vi "editDialog.vi"(0 "reference in":refnum<class "DQMHModuleNode.lvclass">, 1 "insidePackageNode":bool, 5 "error in (no error)":errorcluster) -> (14 "reference out":refnum<class "DQMHModuleNode.lvclass">, 15 "changeConnection":T1, 16 "cancel":bool, 19 "error out":errorcluster)   [LabVIEW 2020, in "DQMHModuleNode.lvclass"]
doc: "Edit Dialog"
uses:
  <resource>/Framework/Providers/Open_GDS/UML/DQMHModuleNode_class/DQMHModuleNode.lvclass
  C:/Program Files (x86)/National Instruments/LabVIEW 2020/resource/Framework/Providers/Open_GDS/UML/AbstractNode_class/AbstractNode.lvclass
  <resource>/Framework/Providers/Open_GDS/UML/AbstractNode_class/private/NodeConnectionStatsType.ctl
  <resource>/Framework/Providers/Open_GDS/UML/UMLEditor/UMLEditor_StoredPathes.ctl
  <resource>/Framework/Providers/Open_GDS/UML/ContextHelp/ContextHelp_HelpTexts.ctl
  <vilib>/LabVIEW Icon API/lv_icon/Classes/Icon/Icon.lvclass
  <vilib>/LabVIEW Icon API/API_Text.ctl
  <vilib>/LabVIEW Icon API/API_Rectangle Colors.ctl
  <vilib>/LabVIEW Icon API/API_Rectangle Dimension.ctl
  <vilib>/LabVIEW Icon API/API_User Layer Data.ctl
  <vilib>/Utility/miscctls.llb/LVPoint32TypeDef.ctl
  <vilib>/picture/picture.llb/imagedata.ctl
  <vilib>/LabVIEW Icon API/API_Test Settings.ctl
  <vilib>/LabVIEW Icon API/lv_icon/Controls/Alignment.ctl
  <vilib>/LabVIEW Icon API/API_Text Colors.ctl
  <resource>/Framework/Providers/Open_GDS/UML/MultiLineString_class/MultiLineString.lvclass
  <resource>/Framework/Providers/Open_GDS/UML/AbstractNode_class/AbstractNode.lvclass
  <resource>/Framework/Providers/Open_GDS/UML/DQMH_API_class/DQMH_API.lvclass
  <vilib>/LabVIEW Icon API/LabVIEW Icon API.lvlib
panel:
  in  "ShowDescription":bool caption="Show Internal Data"
  out "ModuleIcon":picture caption="Library icon"
  in  "ModuleDescription":string caption="Module Description"
  in  "Template":u16(ring) items=["Singleton", "Cloneable"]
  out "RelText":string="Relative path used"
  in  "ShowInternalData":bool caption="Show Internal Data"
  in  "ShowEvents":bool caption="Show Events"
  in  "Help":bool
  in  "AddEvent":bool
  in  "AddInternalData":bool
  in  "Module Name":string
  in  "ModulePath":path caption="Library Path(Optional)"
  in  "InternalData":string caption="Internal Data"
  in  "Events":string
  in  "connection":bool caption="Disconnect from Package"
  in  "Cancel Button":bool
  in  "OK Button":bool
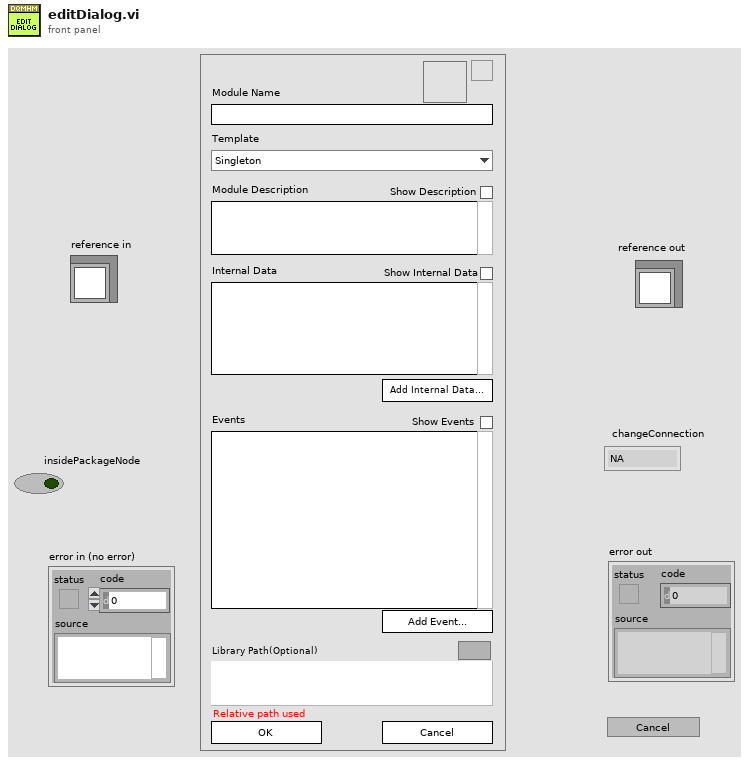
[diagram p1: front panel]
types:
  T1 = typedef "AbstractNode.lvclass/NodeConnectionStatsType.ctl" = enum16{"NA", "Connect", "DisConnect"}
  T2 = cluster{"Cancelled":bool, "Event":refnum<event-registration>, "changeConnection":T1, "Icon":u8[][], "NameModifed":bool}
  T3 = typedef "UMLEditor_StoredPathes.ctl" = enum16{"LastSearchPath", "QueuedArrayStateVI", "ClassBasePath", "ViTemplatePath", "ApplicationTemplatePath", "IniFilePath", "WizDir", "RevPlugInPath"}
  T4 = cluster{"left":i16, "top":i16, "right":i16, "bottom":i16}
  T5 = cluster{"Selection Start":u32, "Selection End":u32}
  T6 = cluster{"LibraryIcon":string, "HeaderRows(1)":u8}
  T7 = typedef "ContextHelp_HelpTexts.ctl" = enum16{"None(Hide)", "Default", "Help", "Welcome", "GettingStarted", "ClassDiagram_Help", "SequenceDiagram_Help", "UseCaseDiagram_Help", "BSelect", "BClass", "BInterface", "BPackage", "BNote", "BDependency", "BInheritance", "BInterfaceImplementation", "BAssociation", "BAggregation", "BCompAggregation", "BNoteConnector", "BObject", "BActionBar", "BCall", "BSystem", "BActor", "BUseCase", "BGeneralization", "BIncludes", "BExtends", "BUseCaseDiagramAssociation", "ClassRelationshipEdge editDialog_Bent Style", "ClassRelationshipEdge editDialog_RelationType", "ClassRelationshipEdge editDialog_Reverse association", "ClassRelationshipEdge editDialog_Start label", "ClassRelationshipEdge editDialog_Middle label", "ClassRelationshipEdge editDialog_End label", "UMLEditor reversedEngineering_Pathes", "ReversedEngineering StateReverseDialog_Help", "ReversedEngineering StateQueuedSettings_Help", "UMLEditor reversedEngineering_AddTopVIs", "UMLEditor reversedEngineering_AddClasses", "UMLEditor reversedEngineering_AddDirs", "UMLEditor reversedEngineering_Recursively", "UMLEditor reversedEngineering_Remove", "UMLEditor reversedEngineering_ClearList", "UMLEditor reversedEngineering_HideSubAss", "UMLEditor reversedEngineering_CreateTypes", "UMLEditor reversedEngineering_OnlyInheritance", "UMLEditor reversedEngineering_CreateApplication", "UMLEditor reversedEngineering_OK", "UMLEditor reversedEngineering_Cancel", "UMLEditor reversedEngineering_Help", "UMLEditor createWizardScriptFile_ScriptfilePath", "UMLEditor createWizardScriptFile_ClassPath", "UMLEditor createWizardScriptFile_Use", "UMLEditor createWizardScriptFile_PrivateDirName", "UMLEditor createWizardScriptFile_DirAppend", "UMLEditor createWizardScriptFile_Separator Character", "UMLEditor createWizardScriptFile_OK", "UMLEditor createWizardScriptFile_Cancel", "UMLEditor createWizardScriptFile_Help", "ClassNode editDialog_Class Name", "InterfaceNode editDialog_Class Name", "ClassNode editDialog_Attribute", "ClassNode editDialog_Methods", "InterfaceNode editDialog_Methods", "ClassNode editDialog_connection", "InterfaceNode editDialog_connection", "ClassNode editDialog_StereoType", "ClassNode editDialog_ShowAttrib", "ClassNode editDialog_ShowMethods", "ClassNode editDialog_ClassPath", "ClassNode editDialog_AddAttribute", "ClassNode editDialog_AddMethod", "InterfaceNode editDialog_AddMethod", "ClassNode AttributeGuide_AttributeName", "ClassNode AttributeGuide_Array?", "ClassNode AttributeGuide_Data Type", "ClassNode AttributeGuide_RefName", "ClassNode AttributeGuide_Preview", "ClassNode AttributeGuide_OK", "ClassNode AttributeGuide_Cancel", "ClassNode MethodGuide_Visibility", "ClassNode MethodGuide_Method Name", "ClassNode MethodGuide_Preview", "ClassNode MethodGuide_OK", "ClassNode MethodGuide_Cancel", "CallNode EditCallProperties_AllButtons", "ObjectNode EditObjectlProperties_AllButtons", "ActorNode EditActorProperties_AllButtons", "UseCaseRelationshipNode EditUseCaselProperties_AllButtons", "UseCaseNode EditUseCaselProperties_AllButtons", "SystemNode EditSystemProperties_AllButtons", "ReversedEngineering UpdateAttributes_AllButtons", "StateNode editDialog_AllButtons", "StateTransition editDialog_AllButtons", "ArrangeNodes Main_Picture", "ArrangeNodes Main_Zoom", "ArrangeNodes Main_Auto Zoom", "ArrangeNodes Main_shorten", "ArrangeNodes Main_Min Length", "ArrangeNodes Main_Max Length", "ArrangeNodes Main_increase", "ArrangeNodes Main_decrease", "ArrangeNodes Main_Shake", "ArrangeNodes Main", "BState", "BInitialState", "BFinalState", "BStateTransition", "StateDiagram_Help", "StateDiagram_PropertiesAllButtons", "ReversedEngineering StateReverseDialog_ClearStates", "ReversedEngineering StateReverseDialog_UseQueuedStateMachines", "ReversedEngineering StateReverseDialog_QueuedSettings", "ReversedEngineering StateReverseDialog_SearchForVIs", "ReversedEngineering StateReverseDialog_SearchCriteria", "OptionsDialog_ClassBasePath", "OptionsDialog_VIPath", "OptionsDialog_ApplicationPath", "OptionsDialog_WizDir", "OptionsDialog_IniFilePath", "OptionsDialog_DefineColors", "OptionsDialog_Help", "OptionsDialog_CreateTypes", "ClassRelationshipEdge editDialog_SplitWire"}
  T8 = typedef "LabVIEW Icon API.lvlib/API_Test Settings.ctl" = cluster{"Font":string, "Alignment":T9, "Size":u8, "Center text":bool, "Capitalize text":bool, "Text color":T10}
  T9 = typedef "Alignment.ctl" = u16
  T10 = typedef "LabVIEW Icon API.lvlib/API_Text Colors.ctl" = cluster{"Line 1 color":u32, "Line 2 color":u32, "Line 3 color":u32, "Line 4 color":u32}
  T11 = typedef "LabVIEW Icon API.lvlib/API_User Layer Data.ctl" = cluster{"Layer name":string, "Origin":T12, "Icon image data":T13}
  T12 = typedef "LVPoint32TypeDef.ctl" = cluster{"Horizontal":i32, "Vertical":i32}
  T13 = typedef "imagedata.ctl" = cluster{"image type":i32, "image depth":i32, "image":u8[], "mask":u8[], "colors":u32[], "Rectangle":cluster{"left":i16, "top":i16, "right":i16, "bottom":i16}}
  T14 = typedef "LabVIEW Icon API.lvlib/API_Rectangle Dimension.ctl" = cluster{"Width":i16, "Height":i16}
  T15 = typedef "LabVIEW Icon API.lvlib/API_Rectangle Colors.ctl" = cluster{"Border":u32, "Background":u32}
  T16 = typedef "LabVIEW Icon API.lvlib/API_Text.ctl" = cluster{"Line 1 text":string, "Line 2 text":string, "Line 3 text":string, "Line 4 text":string}
  T17 = typedef "DQMHModuleNode.lvclass/ObjectAttributes.ctl" = cluster{"DescriptionHeight":dbl, "InternalDataHeight":dbl, "EventsHeight":dbl, "Name":refnum<class "MultiLineString.lvclass">, "Description":refnum<class "MultiLineString.lvclass">, "InternalData":refnum<class "MultiLineString.lvclass">, "Events":refnum<class "MultiLineString.lvclass">, "showDescription":bool, "showInternalData":bool, "showEvents":bool, "DEFAULT_ROUNDING":i32, "DEFAULT_WIDTH":i32, "DEFAULT_HEIGHT":i32, "ClassPath":path, "Template":string, "Icon":u8[][]}
  T18 = typedef "AbstractNode.lvclass/ObjectAttributes.ctl" = cluster{"parent":refnum<class "AbstractNode.lvclass">, "children":refnum<class "AbstractNode.lvclass">[], "Hidden":bool}
  T19 = typedef "ContextHelp_ShowType.ctl" = cluster{"Header":string, "Picture":picture, "Text":string}
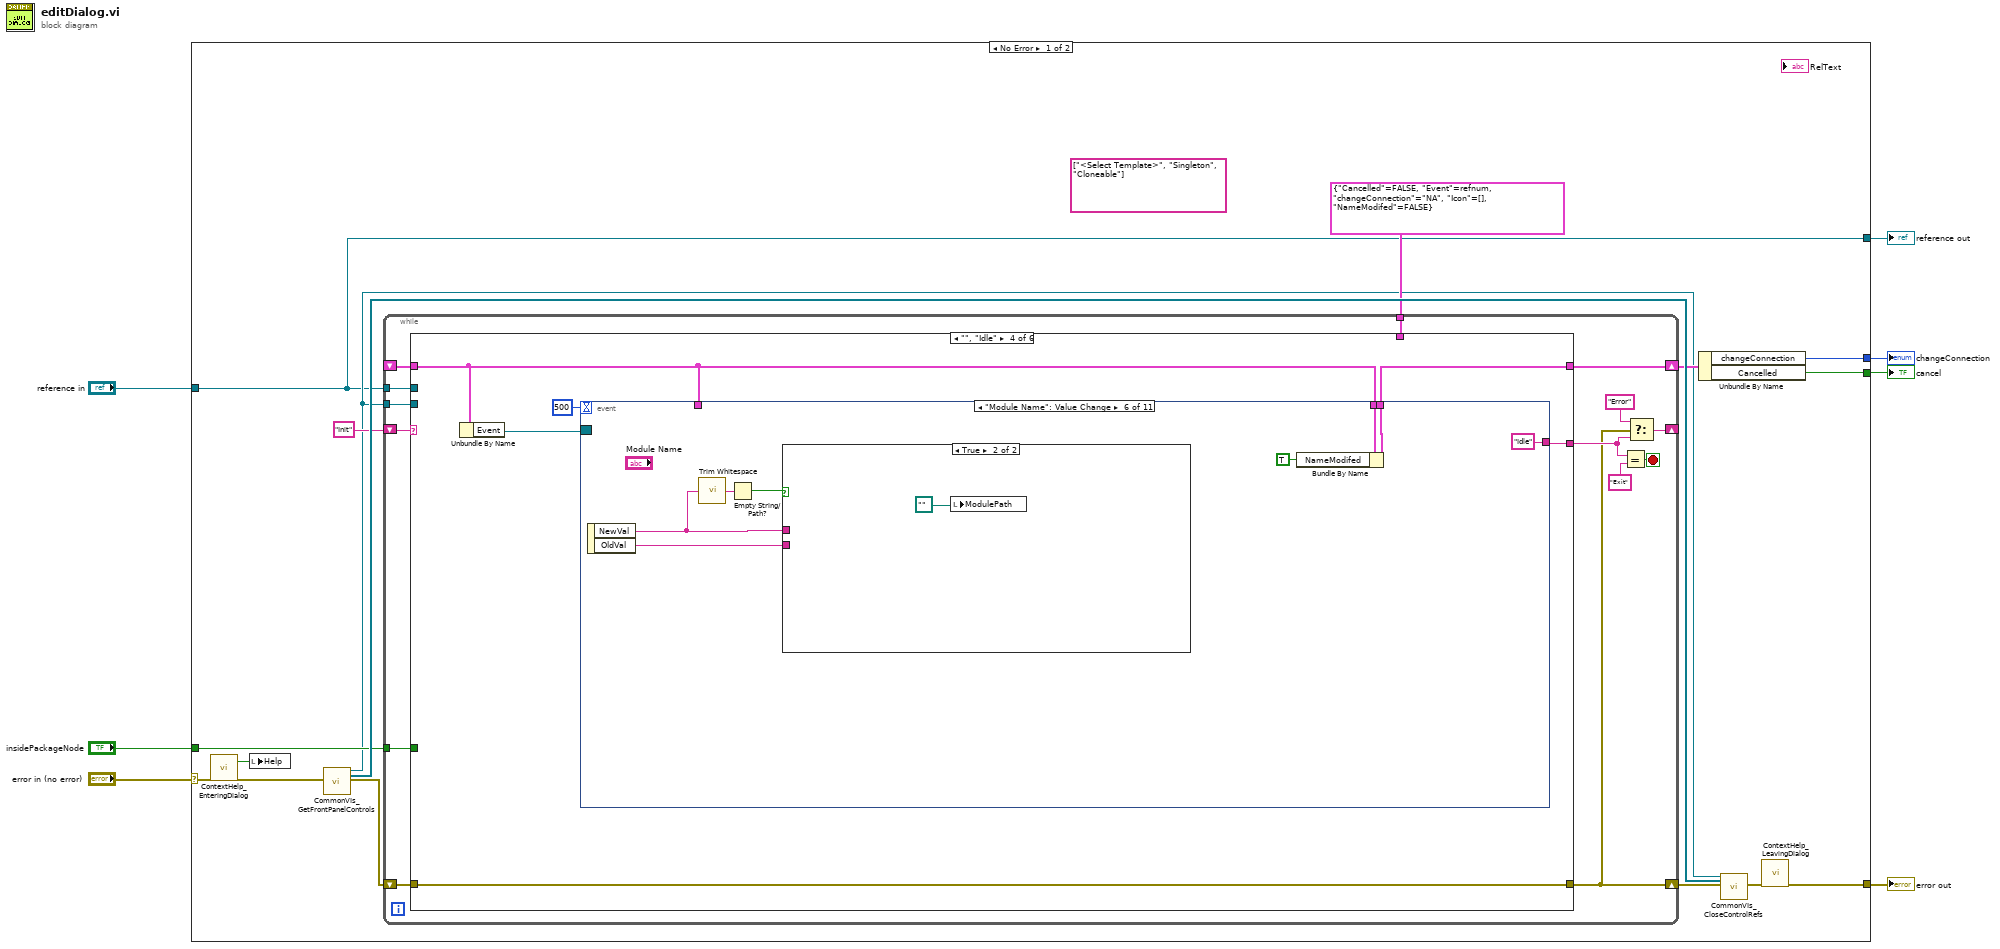
[diagram p0: block diagram]
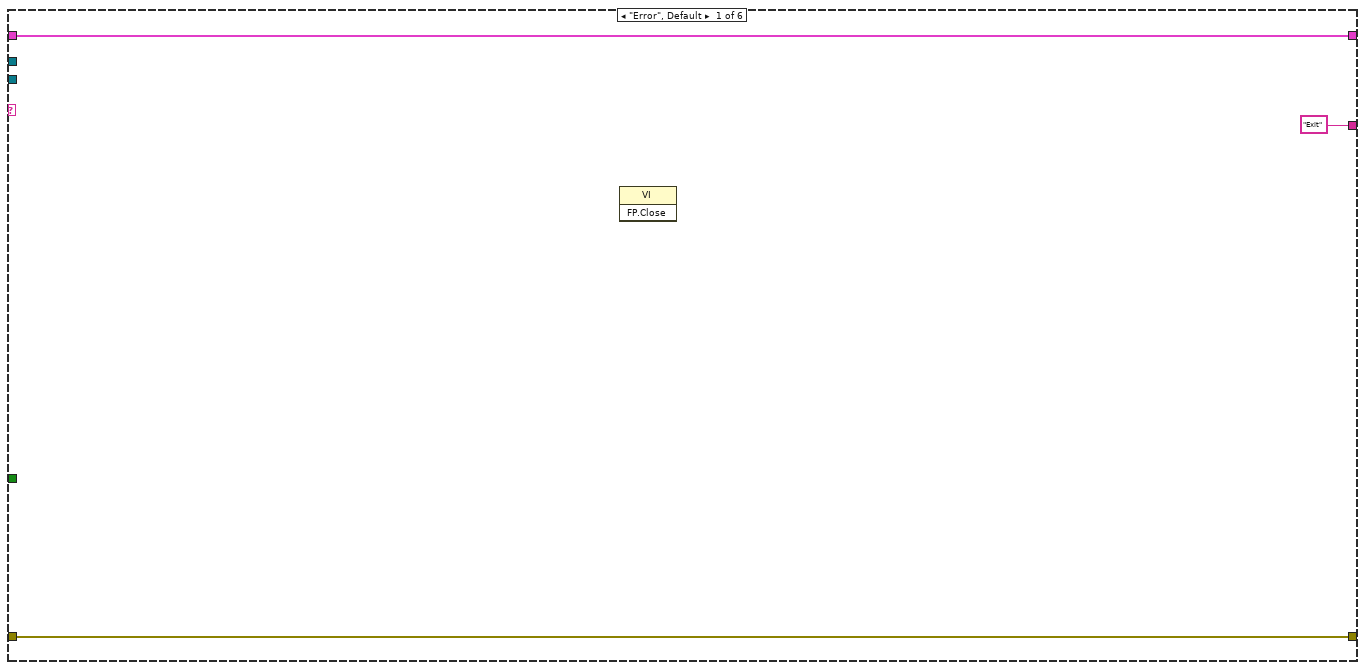
[diagram p2: hidden frame]
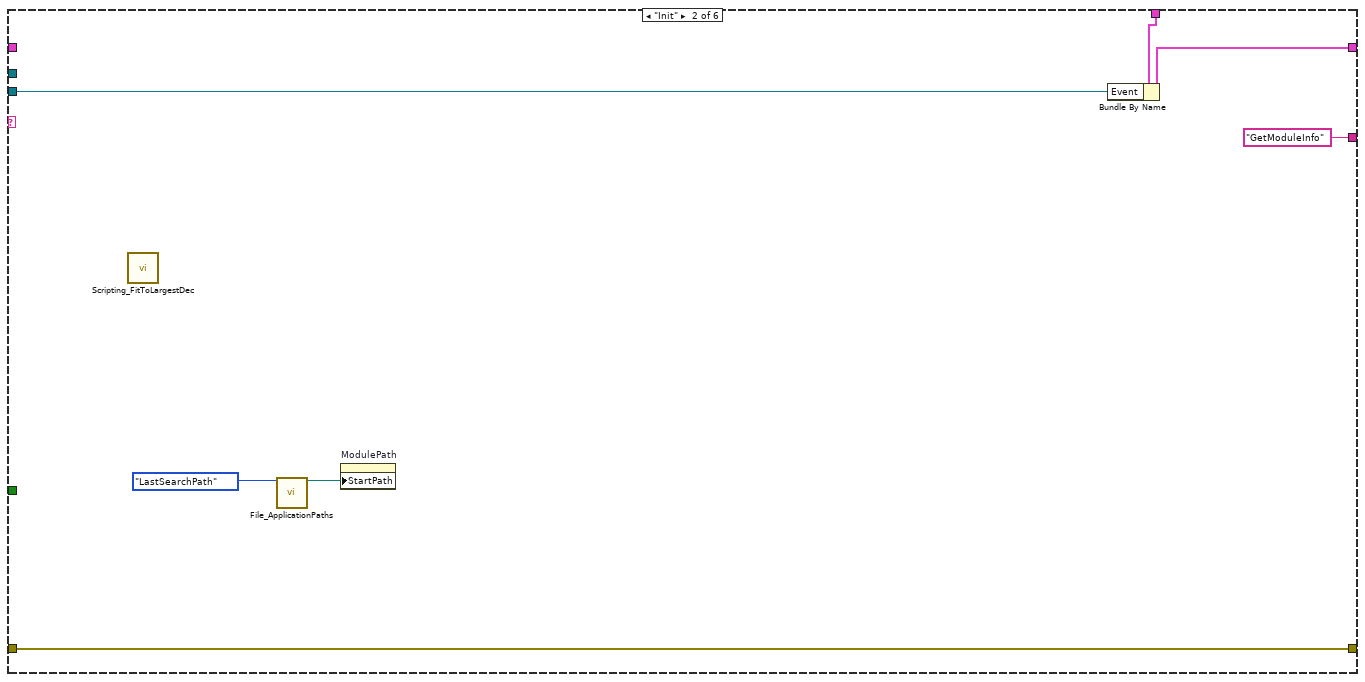
[diagram p3: hidden frame]
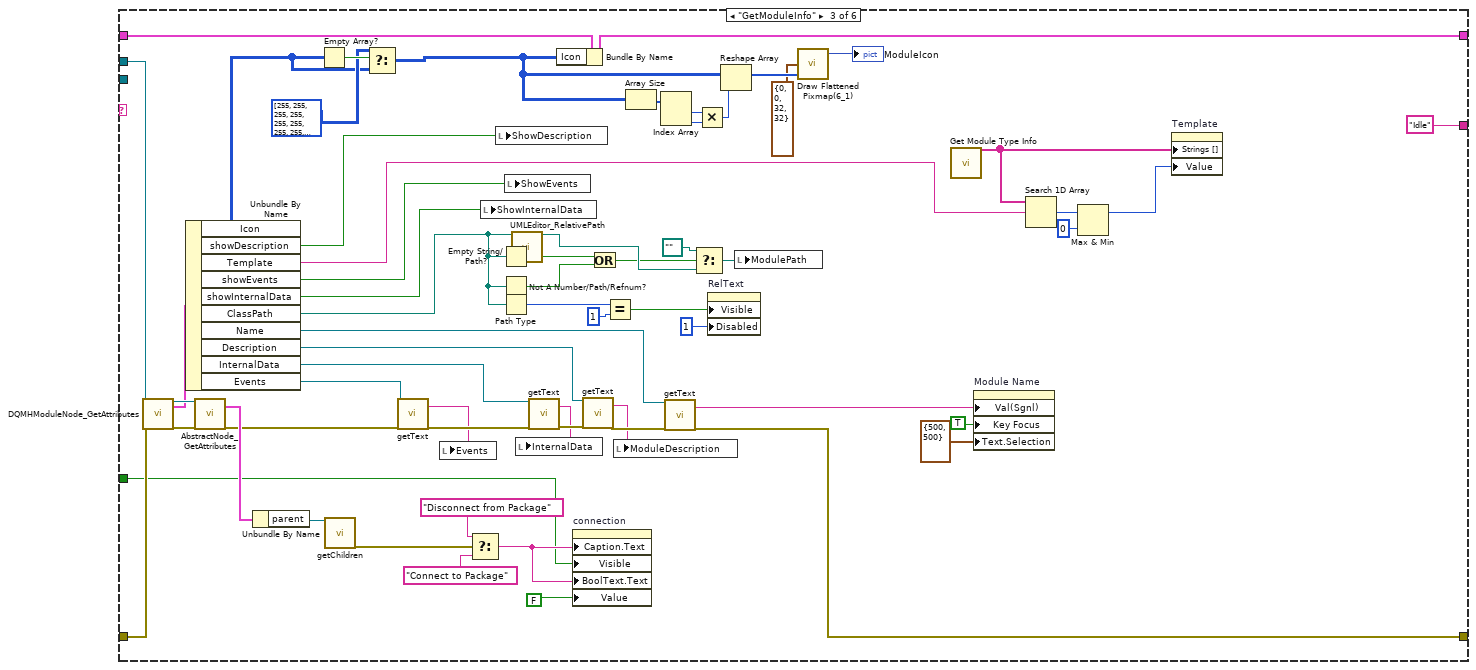
[diagram p4: hidden frame]
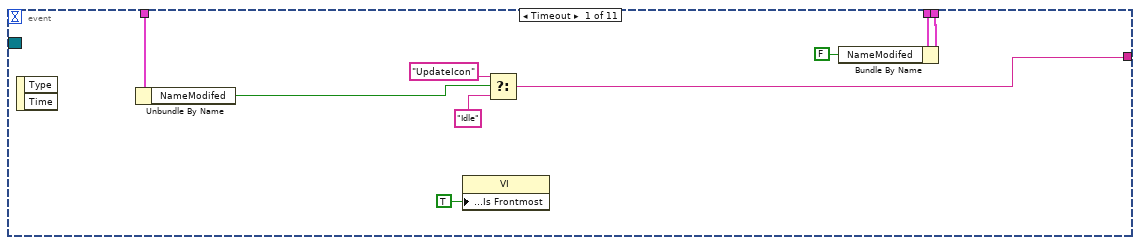
[diagram p5: hidden frame]
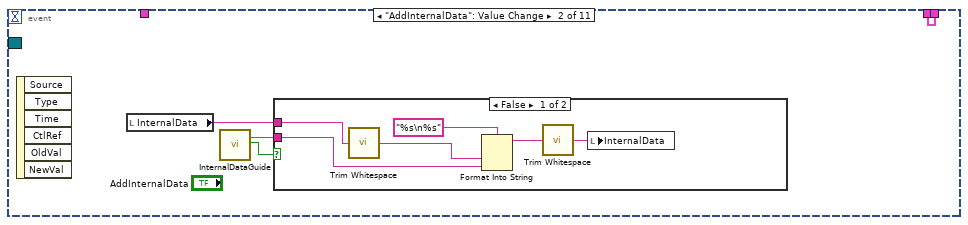
[diagram p6: hidden frame]
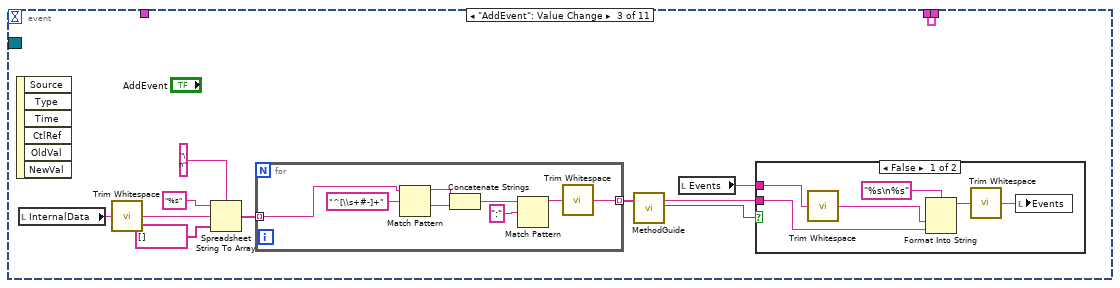
[diagram p8: hidden frame]
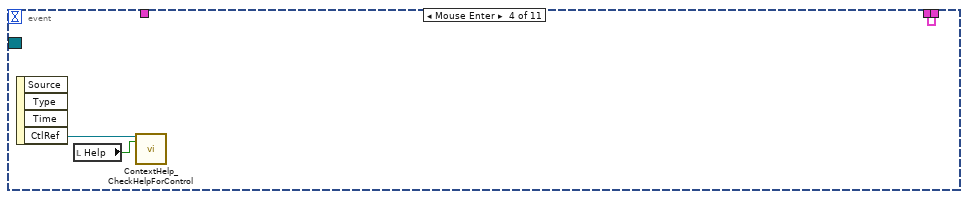
[diagram p10: hidden frame]
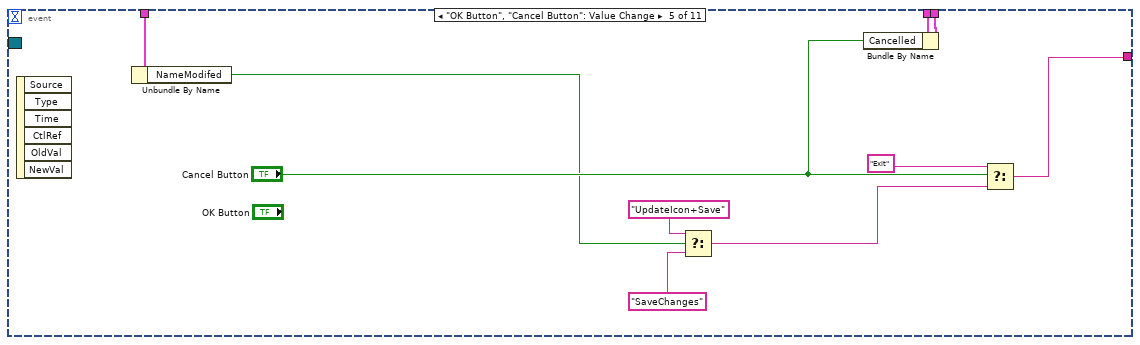
[diagram p11: hidden frame]
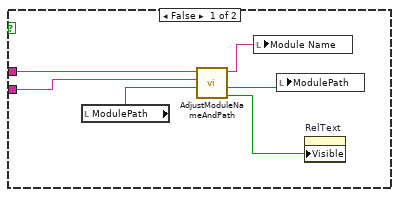
[diagram p12: hidden frame]
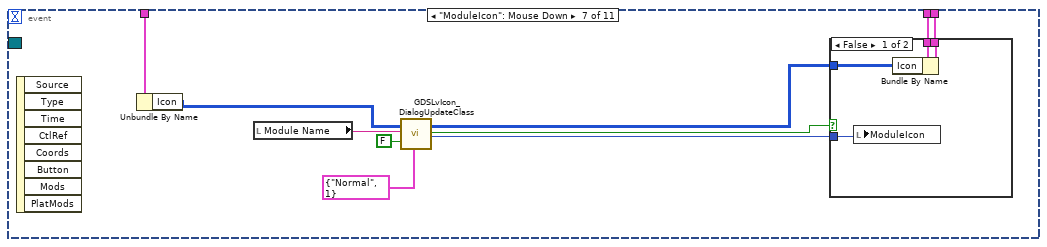
[diagram p13: hidden frame]
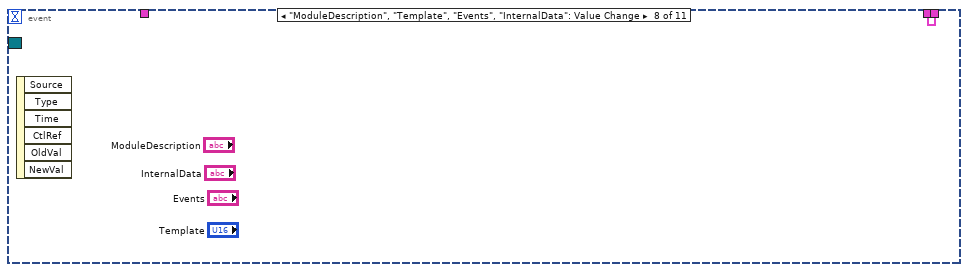
[diagram p15: hidden frame]
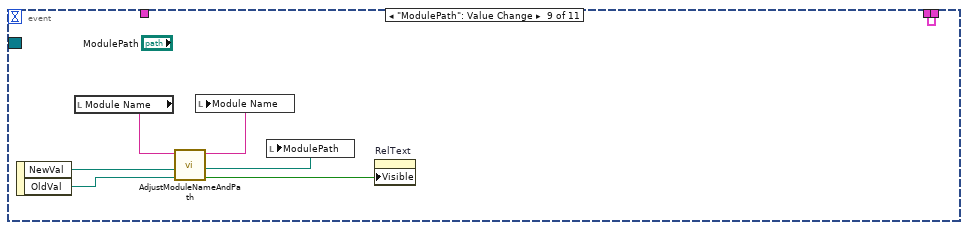
[diagram p16: hidden frame]
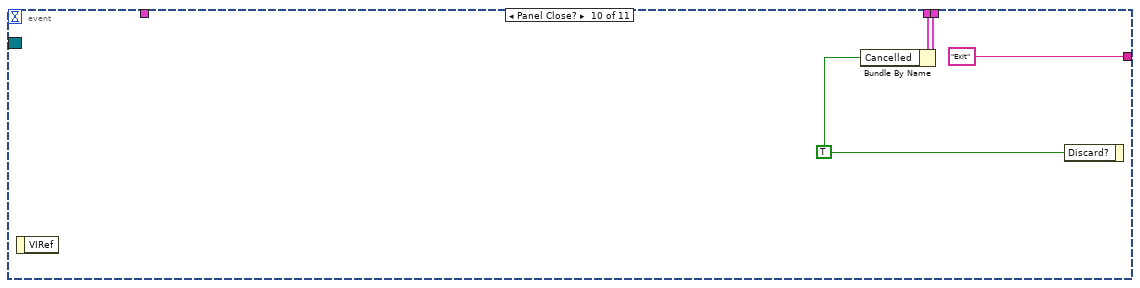
[diagram p17: hidden frame]
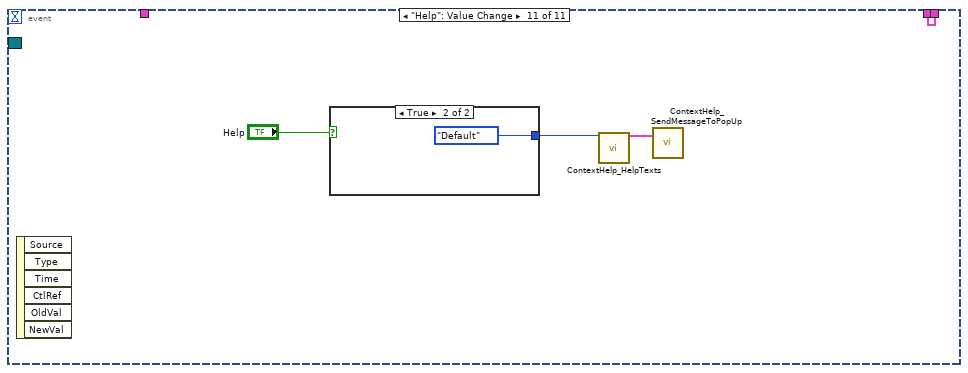
[diagram p18: hidden frame]
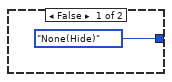
[diagram p19: hidden frame]
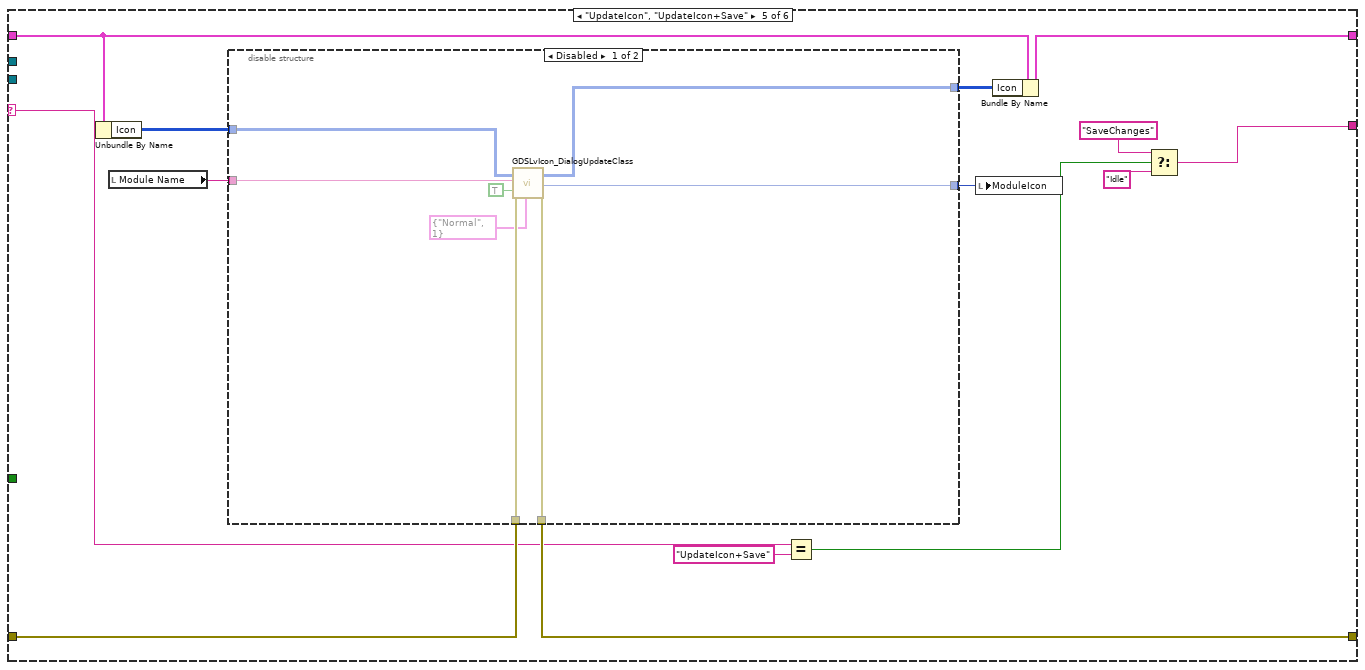
[diagram p20: hidden frame]
diagram:
  n1 = case shown="No Error" "error in (no error)" {
    selector: "error in (no error)" -> [w16 w312]
    tunnel: "reference in" -> [w8 w313]
    tunnel: [w13 w312] -> w5
    tunnel: [w8 w313] -> w4
    tunnel: "insidePackageNode" -> [w17 _]
    tunnel: [w10 _] -> w2
    tunnel: [w9 TRUE ("Key Focus")] -> w1
    frame No Error {
      (unwired) string[] ["<Select Template>", "Singleton", "Cloneable"] ("Strings []")
      n2 = call <resource>:"ContextHelp_EnteringDialog.vi"("error in (no error)"=w16) -> ("HelpStatus"=w23:bool, "error out"=w20:errorcluster)  [unwired: 2 in, 15 out]
      n3 = local write "Help"(w23) -> ()
      n4 = call <resource>:"CommonVIs_GetFrontPanelControls.vi"("error in (no error)"=w20) -> ("Event Registration Refnum"=w11:refnum<event-registration>, "ControlRefs"=w22:refnum<vi>[], "error out"=w15:errorcluster)  [unwired: 1 in, 15 out]
      n5 = while {
        shift-right: [w30] -> w14
        shift-left: w15 -> [w37]
        shift-right: [w35] -> _
        shift-left: "Init" -> [w36]
        shift-right: [w29] -> w12
        shift-left: _ -> [w28]
        tunnel: T2 {"Cancelled"=FALSE, "Event"=refnum, "changeConnection"=enum."NA", "Icon"=[], "NameModifed"=FALSE} -> [w27]
        tunnel: w17 -> [w26]
        tunnel: w11 -> [w25]
        tunnel: w8 -> [w24]
        stop <- w34 stop-if-true
        n6 = case shown="\"\", \"Idle\"" w36 {
          selector: w36 -> [_ _ _ _ w225 _]
          tunnel: w37 -> [w40 w46 w102 w112 w231 w276]
          tunnel: [w40 w46 w69 w112 w232 w266] -> w30
          tunnel: ["Exit" "GetModuleInfo" "Idle" w113 w221 "Exit"] -> w31
          tunnel: [w38 w45 w61 w114 w227 w280] -> w29
          tunnel: w28 -> [w38 _ w108 w109 w230 w261]
          tunnel: w27 -> [_ w44 _ _ _ _]
          tunnel: w26 -> [_ _ w95 _ _ w278]
          tunnel: w25 -> [_ w42 _ _ _ _]
          tunnel: w24 -> [_ _ w81 _ _ w281]
          frame "Error", Default {
            n7 = invoke class="VI" method="FP.Close"() -> ()  [unwired: 3 in, 3 out]
          }
          frame "Init" {
            n8 = call <resource>:"Scripting_FitToLargestDec.vi"() -> ()  [unwired: 6 in, 2 out]
            n9 = call <resource>:"File_ApplicationPaths.vi"("PathName"=UMLEditor_StoredPathes."LastSearchPath" ("UMLPathes")) -> ("Path Out"=w43:path)  [unwired: 3 in, 15 out]
            n10 = property on="ModulePath" class="Path"("StartPath"=w43) -> ()  [unwired: 2 in, 2 out]
            n11 = Bundle By Name(cluster=w44, "Event"=w42) -> (w45:T2)
          }
          frame "GetModuleInfo" {
            n12 = call <resource>:"DQMHModuleNode_GetAttributes.vi"("reference in"=w81, "error in (no error)"=w102) -> ("reference out"=w104:refnum<class "DQMHModuleNode.lvclass">, "Data"=w100:T17, "error out"=w103:errorcluster)  [unwired: 1 in, 14 out]
            n13 = Unbundle By Name(w100) -> ("Icon"=w58:u8[][], "showDescription"=w49:bool, "Template"=w66:string, "showEvents"=w84:bool, "showInternalData"=w83:bool, "ClassPath"=w82:path, "Name"=w99:refnum<class "MultiLineString.lvclass">, "Description"=w98:refnum<class "MultiLineString.lvclass">, "InternalData"=w97:refnum<class "MultiLineString.lvclass">, "Events"=w74:refnum<class "MultiLineString.lvclass">)
            n14 = call <resource>:"AbstractNode_GetAttributes.vi"("reference in"=w104, "error in (no error)"=w103) -> ("Data"=w101:T18, "error out"=w70:errorcluster)  [unwired: 14 in, 2 out]
            n15 = Unbundle By Name(w101) -> ("parent"=w68:refnum<class "AbstractNode.lvclass">)
            n16 = Empty Array?(array=w58) -> (empty?=w60:bool)
            n17 = call-dynamic "getChildren.vi"("reference"=w68) -> ("error out"=w67:errorcluster)  [unwired: 15 in, 3 out]
            n18 = Select(t=u8[][] [[255, 255, 255, 255, 255, 255, 255, 255, 255, 255, 255, 255, 255, 255, 255, 255, 255, 255, 255, 255, 255, 255, 255, 255, 255, 255, 255, 255, 255, 255, 255, 255], [255, 5, 5, 5, 5, 5, 5, 5, 5, 5, 5, 5, 5, 5, 5, 5, 5, 5, 5, 5, 5, 5, 5, 5, 5, 5, 5, 5, 5, 5, 5, 255], [255, 5, 5, 5, 5, 5, 255, 255, 255, 5, 5, 5, 255, 255, 5, 5, 255, 5, 5, 5, 255, 5, 255, 5, 5, 255, 5, 5, 5, 5, 5, 255], [255, 5, 5, 5, 5, 5, 255, 5, 5, 255, 5, 255, 5, 5, 255, 5, 255, 255, 5, 255, 255, 5, 255, 5, 5, 255, 5, 5, 5, 5, 5, 255], [255, 5, 5, 5, 5, 5, 255, 5, 5, 255, 5, 255, 5, 5, 255, 5, 255, 5, 255, 5, 255, 5, 255, 255, 255, 255, 5, 5, 5, 5, 5, 255], [255, 5, 5, 5, 5, 5, 255, 5, 5, 255, 5, 255, 5, 255, 5, 5, 255, 5, 5, 5, 255, 5, 255, 5, 5, 255, 5, 5, 5, 5, 5, 255], [255, 5, 5, 5, 5, 5, 255, 255, 255, 5, 5, 5, 255, 5, 255, 5, 255, 5, 5, 5, 255, 5, 255, 5, 5, 255, 5, 5, 5, 5, 5, 255], [255, 5, 5, 5, 5, 5, 5, 5, 5, 5, 5, 5, 5, 5, 5, 5, 5, 5, 5, 5, 5, 5, 5, 5, 5, 5, 5, 5, 5, 5, 5, 255], [255, 255, 255, 255, 255, 255, 255, 255, 255, 255, 255, 255, 255, 255, 255, 255, 255, 255, 255, 255, 255, 255, 255, 255, 255, 255, 255, 255, 255, 255, 255, 255], [255, 156, 156, 156, 156, 156, 156, 156, 156, 156, 156, 156, 156, 156, 156, 156, 156, 156, 156, 156, 156, 156, 156, 156, 156, 156, 156, 156, 156, 156, 156, 255], [255, 156, 156, 156, 156, 156, 156, 156, 156, 156, 156, 156, 156, 156, 156, 5, 5, 156, 156, 156, 156, 156, 156, 156, 156, 156, 156, 156, 156, 156, 156, 255], [255, 156, 156, 156, 156, 156, 156, 156, 156, 156, 156, 156, 156, 5, 89, 47, 89, 89, 5, 156, 156, 156, 156, 156, 156, 156, 156, 156, 156, 156, 156, 255], [255, 156, 156, 156, 156, 156, 156, 156, 156, 156, 156, 5, 89, 47, 5, 5, 5, 5, 89, 89, 5, 156, 156, 156, 156, 156, 156, 156, 156, 156, 156, 255], [255, 156, 156, 156, 156, 156, 156, 156, 156, 5, 89, 47, 5, 5, 5, 5, 5, 5, 5, 5, 89, 89, 5, 156, 156, 156, 156, 156, 156, 156, 156, 255], [255, 156, 156, 156, 156, 156, 156, 156, 89, 47, 5, 5, 5, 5, 5, 5, 5, 5, 5, 5, 5, 5, 89, 89, 156, 156, 156, 156, 156, 156, 156, 255], [255, 156, 156, 156, 156, 156, 156, 156, 47, 47, 5, 5, 5, 5, 5, 5, 5, 5, 5, 5, 5, 5, 173, 89, 156, 156, 156, 156, 156, 156, 156, 255], [255, 156, 156, 156, 156, 156, 156, 156, 47, 89, 89, 47, 5, 5, 5, 5, 5, 5, 5, 5, 173, 173, 173, 47, 156, 156, 156, 156, 156, 156, 156, 255], [255, 156, 156, 156, 156, 156, 156, 156, 47, 89, 89, 89, 89, 47, 5, 5, 5, 5, 173, 173, 173, 173, 173, 47, 156, 156, 156, 156, 156, 156, 156, 255], [255, 156, 156, 156, 156, 156, 156, 156, 47, 89, 89, 89, 89, 89, 89, 47, 89, 173, 173, 173, 173, 173, 173, 47, 156, 156, 156, 156, 156, 156, 156, 255], [255, 156, 156, 156, 156, 156, 156, 156, 47, 89, 89, 89, 89, 89, 89, 89, 173, 173, 173, 173, 173, 173, 173, 47, 156, 156, 156, 156, 156, 156, 156, 255], [255, 156, 156, 156, 156, 156, 156, 156, 47, 89, 89, 89, 89, 89, 89, 89, 173, 173, 173, 173, 173, 173, 173, 47, 156, 156, 156, 156, 156, 156, 156, 255], [255, 156, 156, 156, 156, 156, 156, 156, 47, 89, 89, 89, 89, 89, 89, 89, 173, 173, 173, 173, 173, 173, 173, 47, 156, 156, 156, 156, 156, 156, 156, 255], [255, 156, 156, 156, 156, 156, 156, 156, 47, 89, 89, 89, 89, 89, 89, 89, 173, 173, 173, 173, 173, 173, 173, 47, 156, 156, 156, 156, 156, 156, 156, 255], [255, 156, 156, 156, 156, 156, 156, 156, 47, 89, 89, 89, 89, 89, 89, 89, 173, 173, 173, 173, 173, 173, 173, 47, 156, 156, 156, 156, 156, 156, 156, 255], [255, 156, 156, 156, 156, 156, 156, 156, 89, 89, 89, 89, 89, 89, 89, 89, 173, 173, 173, 173, 173, 173, 89, 89, 172, 172, 172, 156, 156, 156, 156, 255], [255, 156, 156, 156, 156, 156, 156, 156, 156, 47, 47, 89, 89, 89, 89, 89, 173, 173, 173, 173, 89, 89, 47, 172, 172, 172, 172, 172, 172, 156, 156, 255], [255, 156, 156, 156, 156, 156, 156, 156, 156, 156, 156, 47, 89, 89, 89, 89, 173, 173, 89, 89, 47, 172, 172, 172, 172, 172, 172, 156, 156, 156, 156, 255], [255, 156, 156, 156, 156, 156, 156, 156, 156, 156, 156, 156, 156, 47, 89, 89, 89, 89, 5, 172, 172, 172, 172, 172, 172, 172, 156, 156, 156, 156, 156, 255], [255, 156, 156, 156, 156, 156, 156, 156, 156, 156, 156, 156, 156, 156, 156, 47, 5, 172, 172, 172, 172, 172, 172, 172, 156, 156, 156, 156, 156, 156, 156, 255], [255, 156, 156, 156, 156, 156, 156, 156, 156, 156, 156, 156, 156, 156, 156, 156, 156, 156, 172, 172, 172, 172, 156, 156, 156, 156, 156, 156, 156, 156, 156, 255], [255, 156, 156, 156, 156, 156, 156, 156, 156, 156, 156, 156, 156, 156, 156, 156, 156, 156, 156, 156, 156, 156, 156, 156, 156, 156, 156, 156, 156, 156, 156, 255], [255, 255, 255, 255, 255, 255, 255, 255, 255, 255, 255, 255, 255, 255, 255, 255, 255, 255, 255, 255, 255, 255, 255, 255, 255, 255, 255, 255, 255, 255, 255, 255]] ("flat data"), s=w60, f=w58) -> (s? t:f=w51:u8[][])
            n19 = call-dynamic "getText.vi"("reference"=w74, "error in (no error)"=w70) -> ("text"=w73:string, "error out"=w75:errorcluster)  [unwired: 15 in, 1 out]
            n20 = local write "Events"(w73) -> ()
            n21 = Select(t="Disconnect from Package", s=w67, f="Connect to Package") -> (s? t:f=w107:string)
            n22 = local write "ShowInternalData"(w83) -> ()
            n23 = local write "ShowDescription"(w49) -> ()
            n24 = Empty String/Path?(string/path=w82) -> (empty?=w91:bool)
            n25 = Not A Number/Path/Refnum?(number/path/refnum=w82) -> (NaN/Path/Refnum?=w90:bool)
            n26 = Path Type(1:w82) -> (0:w86:i16)
            n27 = local write "ShowEvents"(w84) -> ()
            n28 = call <resource>:"UMLEditor_RelativePath.vi"("Path In"=w82) -> ("ConvertToAbsolutePath(If possible)"=w94:path)  [unwired: 1 in, 17 out]
            n29 = call-dynamic "getText.vi"("reference"=w97, "error in (no error)"=w75) -> ("text"=w72:string, "error out"=w76:errorcluster)  [unwired: 15 in, 1 out]
            n30 = local write "InternalData"(w72) -> ()
            n31 = Bundle By Name(cluster=w108, "Icon"=w51) -> (w61:T2)
            n32 = property on="connection" class="Bool (strict)"("Caption.Text"=w107, "Visible"=w95, "BoolText.Text"=w107, "Value"=FALSE ("connection")) -> ()  [unwired: 2 in, 2 out]
            n33 = call-dynamic "getText.vi"("reference"=w98, "error in (no error)"=w76) -> ("text"=w71:string, "error out"=w77:errorcluster)  [unwired: 15 in, 1 out]
            n34 = Or(x=w91, y=w90) -> (x .or. y?=w92:bool)
            n35 = Equal?(x=w86, y=i16 1) -> (x = y?=w88:bool)
            n36 = local write "ModuleDescription"(w71) -> ()
            n37 = Array Size(array=w51) -> (size(s)=w53:i32[])
            n38 = Index Array(array=w53) -> (element #1=w55:i32, element #2=w54:i32)  [unwired: 2 in]
            n39 = call-dynamic "getText.vi"("reference"=w99, "error in (no error)"=w77) -> ("text"=w78:string, "error out"=w69:errorcluster)  [unwired: 15 in, 1 out]
            n40 = Select(t=path "", s=w92, f=w94) -> (s? t:f=w89:path)
            n41 = Multiply(x=w55, y=w54) -> (x*y=w56:i32)
            n42 = property on="RelText" class="Str"("Visible"=w88, "Disabled"=u8 1) -> ()  [unwired: 2 in, 2 out]
            n43 = Reshape Array(w51, w56) -> (w57:u8[])
            n44 = local write "ModulePath"(w89) -> ()
            n45 = call <vilib>:"Draw Flattened Pixmap(6_1).vi"("rect"=T4 {"left"=0, "top"=0, "right"=32, "bottom"=32}, "flattened pixmap data"=w57) -> ("new picture"=→"ModuleIcon":picture)  [unwired: 7 in]
            n46 = call <resource>:"Get Module Type Info.vi"() -> ("ModuleTypes"=w48:string[])  [unwired: 14 in, 1 out]
            n47 = property on="Module Name" class="Str"("Val(Sgnl)"=w78, "Key Focus"=TRUE, "Text.Selection"=T5 {"Selection Start"=500, "Selection End"=500}) -> ()  [unwired: 2 in, 2 out]
            n48 = Search 1D Array(1D array=w48, element=w66) -> (index of element=w65:i32)  [unwired: 1 in]
            n49 = Max & Min(x=w65, y=0) -> (max(x,y)=w63:i32)  [unwired: 1 out]
            n50 = property on="Template" class="Ring (strict)"("Strings []"=w48, "Value"=w63) -> ()  [unwired: 2 in, 2 out]
          }
          frame "", "Idle" {
            n51 = Unbundle By Name(w109) -> ("Event"=w111:refnum<event-registration>)
            n52 = event shown="[5] \"Module Name\": Value Change" {
              selector: w111 -> [_ _ _ _ _ _ _ _ _ _ _]
              dyn-events: _ -> [_ _ _ _ _ _ _ _ _ _ _]
              timeout: 500 -> [_ _ _ _ _ _ _ _ _ _ _]
              tunnel: w109 -> [w123 w127 w144 w161 w171 w179 w196 w202 w209 w212 w217]
              tunnel: [w117 w127 w144 w161 w170 w177 w192 w202 w209 w211 w217] -> w114
              tunnel: [w118 _ _ _ w168 "Idle" _ _ _ "Exit" _] -> w113
              tunnel: w109 -> [w121 _ _ _ w166 _ w189 _ _ _ _]
              event Timeout {
                n53 = event-data() -> ()  [unwired: 1 in, 2 out]
                n54 = Unbundle By Name(w121) -> ("NameModifed"=w115:bool)
                n55 = property class="VI"("Front Panel Window:Is Frontmost"=TRUE) -> ()  [unwired: 2 in, 2 out]
                n56 = Select(t="UpdateIcon", s=w115, f="Idle") -> (s? t:f=w118:string)
                n57 = Bundle By Name(cluster=w123, "NameModifed"=FALSE) -> (w117:T2)
              }
              event "AddInternalData": Value Change {
                n58 = event-data() -> ()  [unwired: 1 in, 6 out]
                n59 = local read "InternalData"() -> (w125:string)
                n60 = call <resource>:"InternalDataGuide.vi"() -> ("Preview"=w126:string, "Canceled"=w124:bool)  [unwired: 18 out]
                n61 = case shown="False" w124 {
                  tunnel: w125 -> [w133 _]
                  tunnel: w126 -> [w130 _]
                  frame False {
                    n62 = call <vilib>:"Trim Whitespace.vi"("string"=w133) -> ("trimmed string"=w131:string)  [unwired: 1 in]
                    n63 = Format Into String(format string="%s\n%s", w131, w130) -> (resulting string=w129:string)  [unwired: 2 in, 1 out]
                    n64 = call <vilib>:"Trim Whitespace.vi"("string"=w129) -> ("trimmed string"=w128:string)  [unwired: 1 in]
                    n65 = local write "InternalData"(w128) -> ()
                  }
                  frame True {
                  }
                }
              }
              event "AddEvent": Value Change {
                n66 = event-data() -> ()  [unwired: 1 in, 6 out]
                n67 = local read "InternalData"() -> (w137:string)
                n68 = call <vilib>:"Trim Whitespace.vi"("string"=w137) -> ("trimmed string"=w138:string)  [unwired: 1 in]
                n69 = Spreadsheet String To Array(delimiter (Tab)="\n", format string="%s", spreadsheet string=w138, array type (2D Dbl)=string[] [] ("Attributes")) -> (array=w142:string[])
                n70 = for {
                  tunnel: w142 -> [w152] mode=indexing
                  tunnel: [w148] -> w143 mode=indexing
                  n71 = Match Pattern(string=w152, regular expression="^[\\s+#-]+") -> (before substring=w150:string, after substring=w149:string)  [unwired: 1 in, 2 out]
                  n72 = Concatenate Strings(w150, w149) -> (w146:string)
                  n73 = Match Pattern(string=w146, regular expression=":") -> (before substring=w145:string)  [unwired: 1 in, 3 out]
                  n74 = call <vilib>:"Trim Whitespace.vi"("string"=w145) -> ("trimmed string"=w148:string)  [unwired: 1 in]
                }
                n75 = call <resource>:"MethodGuide.vi"("Attributes"=w143) -> ("Preview"=w135:string, "Canceled"=w136:bool)  [unwired: 17 out]
                n76 = local read "Events"() -> (w134:string)
                n77 = case shown="False" w136 {
                  tunnel: w134 -> [w158 _]
                  tunnel: w135 -> [w155 _]
                  frame False {
                    n78 = call <vilib>:"Trim Whitespace.vi"("string"=w158) -> ("trimmed string"=w156:string)  [unwired: 1 in]
                    n79 = Format Into String(format string="%s\n%s", w156, w155) -> (resulting string=w154:string)  [unwired: 2 in, 1 out]
                    n80 = call <vilib>:"Trim Whitespace.vi"("string"=w154) -> ("trimmed string"=w153:string)  [unwired: 1 in]
                    n81 = local write "Events"(w153) -> ()
                  }
                  frame True {
                  }
                }
              }
              event Mouse Enter {
                n82 = event-data() -> ("CtlRef"=w159:refnum<vi>)  [unwired: 1 in, 3 out]
                n83 = local read "Help"() -> (w160:bool)
                n84 = call <resource>:"ContextHelp_CheckHelpForControl.vi"("Ctl Refnum"=w159, "Help"=w160) -> ()  [unwired: 1 in, 17 out]
              }
              event "OK Button", "Cancel Button": Value Change {
                n85 = event-data() -> ()  [unwired: 1 in, 6 out]
                n86 = Unbundle By Name(w166) -> ("NameModifed"=w165:bool)
                n87 = Select(t="UpdateIcon+Save" ("y"), s=w165, f="SaveChanges") -> (s? t:f=w163:string)
                n88 = Bundle By Name(cluster=w171, "Cancelled"="Cancel Button") -> (w170:T2)
                n89 = Select(t="Exit", s="Cancel Button", f=w163) -> (s? t:f=w168:string)
              }
              event "Module Name": Value Change {
                n90 = event-data() -> ("NewVal"=w174:string, "OldVal"=w175:string)  [unwired: 1 in]
                n91 = call <vilib>:"Trim Whitespace.vi"("string"=w174) -> ("trimmed string"=w172:string)  [unwired: 1 in]
                n92 = Empty String/Path?(string/path=w172) -> (empty?=w173:bool)
                n93 = case shown="True" w173 {
                  tunnel: w175 -> [w185 _]
                  tunnel: w174 -> [w180 _]
                  frame False {
                    n94 = local read "ModulePath"() -> (w182:path)
                    n95 = call <resource>:"AdjustModuleNameAndPath.vi"("NewModulePath"=w182, "OldModuleName"=w185, "NewModuleName"=w180) -> ("RelativePath"=w183:bool, "ModulePath"=w184:path, "ModuleNameOut"=w181:string)  [unwired: 6 in]
                    n96 = local write "Module Name"(w181) -> ()
                    n97 = local write "ModulePath"(w184) -> ()
                    n98 = property on="RelText" class="Str"("Visible"=w183) -> ()  [unwired: 2 in, 2 out]
                  }
                  frame True {
                    n99 = local write "ModulePath"(path "" ("ModulePath")) -> ()
                  }
                }
                n100 = Bundle By Name(cluster=w179, "NameModifed"=TRUE) -> (w177:T2)
              }
              event "ModuleIcon": Mouse Down {
                n101 = event-data() -> ()  [unwired: 1 in, 8 out]
                n102 = Unbundle By Name(w189) -> ("Icon"=w188:u8[][])
                n103 = local read "Module Name"() -> (w194:string)
                n104 = call <resource>:"GDSLvIcon_DialogUpdateClass.vi"("ClassPath(FilePath/ProjectTreePath/LvCLassRef)"=w188, "ClassName"=w194, "AutoUpdate"=FALSE, "LibraryIcon"=T6 {"LibraryIcon"="Normal", "HeaderRows(1)"=1}) -> ("WholeIconOut"=w191:u8[][], "Cancelled"=w190:bool, "IconPictureOut"=w193:picture)  [unwired: 12 in, 1 out]
                n105 = case shown="False" w190 {
                  tunnel: w196 -> [w200 w201]
                  tunnel: w193 -> [w199 _]
                  tunnel: [w198 w201] -> w192
                  tunnel: w191 -> [w197 _]
                  frame False {
                    n106 = local write "ModuleIcon"(w199) -> ()
                    n107 = Bundle By Name(cluster=w200, "Icon"=w197) -> (w198:T2)
                  }
                  frame True {
                  }
                }
              }
              event "ModuleDescription", "Template", "Events", "InternalData": Value Change {
                n108 = event-data() -> ()  [unwired: 1 in, 6 out]
              }
              event "ModulePath": Value Change {
                n109 = event-data() -> ("NewVal"=w208:path, "OldVal"=w207:path)  [unwired: 1 in]
                n110 = local read "Module Name"() -> (w205:string)
                n111 = call <resource>:"AdjustModuleNameAndPath.vi"("OldModulePath"=w207, "NewModulePath"=w208, "NewModuleName"=w205) -> ("RelativePath"=w204:bool, "ModulePath"=w203:path, "ModuleNameOut"=w206:string)  [unwired: 6 in]
                n112 = local write "Module Name"(w206) -> ()
                n113 = local write "ModulePath"(w203) -> ()
                n114 = property on="RelText" class="Str"("Visible"=w204) -> ()  [unwired: 2 in, 2 out]
              }
              event Panel Close? {
                w210 = TRUE ("Discard?")
                n115 = event-data() -> ()  [unwired: 1 in, 1 out]
                n116 = Bundle By Name(cluster=w212, "Cancelled"=w210) -> (w211:T2)
                n117 = event-data("Discard?"=w210) -> ()  [unwired: 1 in, 1 out]
              }
              event "Help": Value Change {
                n118 = event-data() -> ()  [unwired: 1 in, 6 out]
                n119 = case shown="True" "Help" {
                  tunnel: [ContextHelp_HelpTexts."None(Hide)" ("HelpText") ContextHelp_HelpTexts."Default" ("HelpText")] -> w215
                  frame False {
                  }
                  frame True {
                  }
                }
                n120 = call <resource>:"ContextHelp_HelpTexts.vi"("HelpText (enum or string)"=w215) -> ("HelpOut"=w214:T19)  [unwired: 18 out]
                n121 = call <resource>:"ContextHelp_SendMessageToPopUp.vi"("PopUpMessage"=w214) -> ()  [unwired: 2 in, 17 out]
              }
            }
          }
          frame "UpdateIcon", "UpdateIcon+Save" {
            n122 = Unbundle By Name(w230) -> ("Icon"=w229:u8[][])
            n123 = local read "Module Name"() -> (w233:string)
            n124 = disable-structure shown="Disabled" {
              disable-tunnel: w233 -> [w240 w245]
              disable-tunnel: [w239 w246] -> w232
              disable-tunnel: w231 -> [w238 w246]
              disable-tunnel: w229 -> [w237 _]
              disable-tunnel: [w235 w244] -> w228
              disable-tunnel: [w234 w242] -> w226
              frame Disabled {
                n125 = call <resource>:"GDSLvIcon_DialogUpdateClass.vi"("ClassPath(FilePath/ProjectTreePath/LvCLassRef)"=w237, "ClassName"=w240, "AutoUpdate"=TRUE, "error in (no error)"=w238, "LibraryIcon"=T6 {"LibraryIcon"="Normal", "HeaderRows(1)"=1}) -> ("WholeIconOut"=w234:u8[][], "IconPictureOut"=w235:picture, "error out"=w239:errorcluster)  [unwired: 11 in, 1 out]
              }
              frame Enabled {
                n126 = Build Array(T11 {"Layer name"="Banner", "Origin"={"Horizontal"=0, "Vertical"=0}, "Icon image data"={"image type"=0, "image depth"=24, "image"=[0, 0, 0, 0, 0, 0, 0, 0, 0, 0, 0, 0, 0, 0, 0, 0, 0, 0, 0, 0, 0, 0, 0, 0, 0, 0, 0, 0, 0, 0, 0, 0, 0, 0, 0, 0, 0, 0, 0, 0, 0, 0, 0, 0, 0, 0, 0, 0, 0, 0, 0, 0, 0, 0, 0, 0, 0, 0, 0, 0, 0, 0, 0, 0, 0, 0, 0, 0, 0, 0, 0, 0, 0, 0, 0, 0, 0, 0, 0, 0, 0, 0, 0, 0, 0, 0, 0, 0, 0, 0, 0, 0, 0, 0, 0, 0, 0, 0, 0, 255, 255, 255, 255, 255, 255, 255, 255, 255, 255, 255, 255, 255, 255, 255, 255, 255, 255, 255, 255, 255, 255, 255, 255, 255, 255, 255, 255, 255, 255, 255, 255, 255, 255, 255, 255, 255, 255, 255, 255, 255, 255, 255, 255, 255, 255, 255, 255, 255, 255, 255, 255, 255, 255, 255, 255, 255, 255, 255, 255, 255, 255, 255, 255, 255, 255, 255, 255, 255, 255, 255, 255, 255, 255, 255, 255, 255, 255, 255, 255, 255, 255, 255, 255, 255, 255, 255, 255, 255, 255, 0, 0, 0, 0, 0, 0, 255, 255, 255, 255, 255, 255, 255, 255, 255, 255, 255, 255, 255, 255, 255, 255, 255, 255, 255, 255, 255, 255, 255, 255, 255, 255, 255, 255, 255, 255, 255, 255, 255, 255, 255, 255, 255, 255, 255, 255, 255, 255, 255, 255, 255, 255, 255, 255, 255, 255, 255, 255, 255, 255, 255, 255, 255, 255, 255, 255, 255, 255, 255, 255, 255, 255, 255, 255, 255, 255, 255, 255, 255, 255, 255, 255, 255, 255, 255, 255, 255, 255, 255, 255, 255, 255, 255, 255, 255, 255, 0, 0, 0, 0, 0, 0, 255, 255, 255, 255, 255, 255, 255, 255, 255, 255, 255, 255, 255, 255, 255, 255, 255, 255, 255, 255, 255, 255, 255, 255, 255, 255, 255, 255, 255, 255, 255, 255, 255, 255, 255, 255, 255, 255, 255, 255, 255, 255, 255, 255, 255, 255, 255, 255, 255, 255, 255, 255, 255, 255, 255, 255, 255, 255, 255, 255, 255, 255, 255, 255, 255, 255, 255, 255, 255, 255, 255, 255, 255, 255, 255, 255, 255, 255, 255, 255, 255, 255, 255, 255, 255, 255, 255, 255, 255, 255, 0, 0, 0, 0, 0, 0, 255, 255, 255, 255, 255, 255, 255, 255, 255, 255, 255, 255, 255, 255, 255, 255, 255, 255, 255, 255, 255, 255, 255, 255, 255, 255, 255, 255, 255, 255, 255, 255, 255, 255, 255, 255, 255, 255, 255, 255, 255, 255, 255, 255, 255, 255, 255, 255, 255, 255, 255, 255, 255, 255, 255, 255, 255, 255, 255, 255, 255, 255, 255, 255, 255, 255, 255, 255, 255, 255, 255, 255, 255, 255, 255, 255, 255, 255, 255, 255, 255, 255, 255, 255, 255, 255, 255, 255, 255, 255, 0, 0, 0, 0, 0, 0, 255, 255, 255, 255, 255, 255, 255, 255, 255, 255, 255, 255, 255, 255, 255, 255, 255, 255, 255, 255, 255, 255, 255, 255, 255, 255, 255, 255, 255, 255, 255, 255, 255, 255, 255, 255, 255, 255, 255, 255, 255, 255, 255, 255, 255, 255, 255, 255, 255, 255, 255, 255, 255, 255, 255, 255, 255, 255, 255, 255, 255, 255, 255, 255, 255, 255, 255, 255, 255, 255, 255, 255, 255, 255, 255, 255, 255, 255, 255, 255, 255, 255, 255, 255, 255, 255, 255, 255, 255, 255, 0, 0, 0, 0, 0, 0, 255, 255, 255, 255, 255, 255, 255, 255, 255, 255, 255, 255, 255, 255, 255, 255, 255, 255, 255, 255, 255, 255, 255, 255, 255, 255, 255, 255, 255, 255, 255, 255, 255, 255, 255, 255, 255, 255, 255, 255, 255, 255, 255, 255, 255, 255, 255, 255, 255, 255, 255, 255, 255, 255, 255, 255, 255, 255, 255, 255, 255, 255, 255, 255, 255, 255, 255, 255, 255, 255, 255, 255, 255, 255, 255, 255, 255, 255, 255, 255, 255, 255, 255, 255, 255, 255, 255, 255, 255, 255, 0, 0, 0, 0, 0, 0, 255, 255, 255, 255, 255, 255, 255, 255, 255, 255, 255, 255, 255, 255, 255, 255, 255, 255, 255, 255, 255, 255, 255, 255, 255, 255, 255, 255, 255, 255, 255, 255, 255, 255, 255, 255, 255, 255, 255, 255, 255, 255, 255, 255, 255, 255, 255, 255, 255, 255, 255, 255, 255, 255, 255, 255, 255, 255, 255, 255, 255, 255, 255, 255, 255, 255, 255, 255, 255, 255, 255, 255, 255, 255, 255, 255, 255, 255, 255, 255, 255, 255, 255, 255, 255, 255, 255, 255, 255, 255, 0, 0, 0, 0, 0, 0, 0, 0, 0, 0, 0, 0, 0, 0, 0, 0, 0, 0, 0, 0, 0, 0, 0, 0, 0, 0, 0, 0, 0, 0, 0, 0, 0, 0, 0, 0, 0, 0, 0, 0, 0, 0, 0, 0, 0, 0, 0, 0, 0, 0, 0, 0, 0, 0, 0, 0, 0, 0, 0, 0, 0, 0, 0, 0, 0, 0, 0, 0, 0, 0, 0, 0, 0, 0, 0, 0, 0, 0, 0, 0, 0, 0, 0, 0, 0, 0, 0, 0, 0, 0, 0, 0, 0, 0, 0, 0, 0, 0, 0], "mask"=[], "colors"=[], "Rectangle"={"left"=0, "top"=0, "right"=32, "bottom"=9}}} ("User Layer data")) -> (w249:T11[])
                n127 = Bundle By Name(cluster=T16 {"Line 1 text"="", "Line 2 text"="", "Line 3 text"="", "Line 4 text"=""} ("Text"), "Line 1 text"=w245) -> (w256:T16)
                n128 = call <vilib>:"Generate LV Icon User Layers.vi"("User layers"=w249, "Icon in"=refnum<class "Icon.lvclass"> refnum ("Icon.lvclass in")) -> ("error out"=w250:errorcluster, "Icon out"=w251:refnum<class "Icon.lvclass">)  [unwired: 8 in]
                n129 = call <vilib>:"Generate LV Icon Text Layer.vi"("Rectangle colors (black, white)"=T15 {"Border"=0, "Background"=16711422}, "Rectangle dimension (32,32)"=T14 {"Width"=0, "Height"=0}, "error in (no error)"=w250, "Text settings"=T8 {"Font"="Small Fonts", "Alignment"=1, "Size"=8, "Center text"=TRUE, "Capitalize text"=TRUE, "Text color"={"Line 1 color"=0, "Line 2 color"=0, "Line 3 color"=0, "Line 4 color"=0}}, "Text"=w256, "Icon in"=w251) -> ("error out"=w253:errorcluster, "Icon out"=w258:refnum<class "Icon.lvclass">)  [unwired: 4 in]
                n130 = call <vilib>:"Get Flattened Image.vi"("error in (no error)"=w253, "lv_icon.lvlib:Icon.lvclass in"=w258) -> ("Color Image"=w243:T13)  [unwired: 6 in, 3 out]
                n131 = call <vilib>:"Unflatten Pixmap.vi"("image data"=w243) -> ("8-bit pixmap"=w242:u8[][])  [unwired: 4 in, 6 out]
                n132 = call <vilib>:"Draw Flattened Pixmap.vi"("image data"=w243) -> ("new picture"=w244:picture)  [unwired: 8 in]
              }
            }
            n133 = Equal?(x=w225, y="UpdateIcon+Save") -> (x = y?=w223:bool)
            n134 = local write "ModuleIcon"(w228) -> ()
            n135 = Bundle By Name(cluster=w230, "Icon"=w226) -> (w227:T2)
            n136 = Select(t="SaveChanges", s=w223, f="Idle") -> (s? t:f=w221:string)
          }
          frame "SaveChanges" {
            n137 = call <resource>:"DQMHModuleNode_GetAttributes.vi"("reference in"=w281, "error in (no error)"=w276) -> ("Data"=w275:T17, "DataRef"=w291:refnum<data-value>, "error out"=w270:errorcluster)  [unwired: 14 in, 1 out]
            n138 = Unbundle By Name(w275) -> ("Name"=w274:refnum<class "MultiLineString.lvclass">, "Description"=w273:refnum<class "MultiLineString.lvclass">, "InternalData"=w272:refnum<class "MultiLineString.lvclass">, "Events"=w267:refnum<class "MultiLineString.lvclass">)
            n139 = local read "Events"() -> (w268:string)
            n140 = local read "ModuleDescription"() -> (w283:string)
            n141 = local read "Module Name"() -> (w290:string)
            n142 = local read "InternalData"() -> (w282:string)
            n143 = call <vilib>:"Trim Whitespace.vi"("string"=w268) -> ("trimmed string"=w269:string)  [unwired: 1 in]
            n144 = local read "Template"() -> (w262:u16)
            n145 = property on="Template" class="Ring (strict)"() -> ("Strings []"=w264:string[])  [unwired: 2 in, 2 out]
            n146 = case shown="True" "connection" {
              tunnel: [enum16{"NA", "Connect", "DisConnect"}."NA" ("changeConnection") w309] -> w279
              tunnel: w278 -> [_ w310]
              frame False {
              }
              frame True {
                n147 = Select(t=NodeConnectionStatsType."DisConnect" ("changeConnection"), s=w310, f=NodeConnectionStatsType."Connect" ("changeConnection")) -> (s? t:f=w309:T1)
              }
            }
            n148 = call-dynamic "setText.vi"("reference"=w267, "text"=w269, "error in (no error)"=w270) -> ("error out"=w271:errorcluster)  [unwired: 15 in, 1 out]
            n149 = call <vilib>:"Trim Whitespace.vi"("string"=w282) -> ("trimmed string"=w288:string)  [unwired: 1 in]
            n150 = call <vilib>:"Trim Whitespace.vi"("string"=w290) -> ("trimmed string"=w289:string)  [unwired: 1 in]
            n151 = case shown="0, Default" w262 {
              selector: w262 -> [_ w296]
              tunnel: w264 -> [_ w297]
              tunnel: [_ w295] -> w263
              frame 0, Default {
              }
              frame 1.. {
                n152 = Index Array(array=w297, index=w296) -> (element=w295:string)
              }
            }
            n153 = call-dynamic "setText.vi"("reference"=w272, "text"=w288, "error in (no error)"=w271) -> ("error out"=w285:errorcluster)  [unwired: 15 in, 1 out]
            n154 = call <vilib>:"Trim Whitespace.vi"("string"=w283) -> ("trimmed string"=w287:string)  [unwired: 1 in]
            n155 = call-dynamic "setText.vi"("reference"=w273, "text"=w287, "error in (no error)"=w285) -> ("error out"=w284:errorcluster)  [unwired: 15 in, 1 out]
            n156 = call-dynamic "setText.vi"("reference"=w274, "text"=w289, "error in (no error)"=w284) -> ("error out"=w266:errorcluster)  [unwired: 15 in, 1 out]
            n157 = Unbundle By Name(w261) -> ("Icon"=w260:u8[][])
            n158 = local read "ModulePath"() -> (w265:path)
            n159 = call <resource>:"UMLEditor_RelativePath.vi"("Path In"=w265) -> ("ConvertToRelativePath(If possible)"=w292:path)  [unwired: 1 in, 17 out]
            n160 = in-place {
              in-place-border: w292 -> [w301]
              in-place-border: "ShowEvents" -> [w304]
              in-place-border: "ShowInternalData" -> [w303]
              in-place-border: w263 -> [w300]
              in-place-border: w260 -> [w299]
              in-place-border: "ShowDescription" -> [w298]
              n161 = in-place-dvr #1(w291) -> (w305:T17)  [unwired: 1 out]
              n162 = Bundle By Name(cluster=w305, "showDescription"=w298, "showEvents"=w304, "showInternalData"=w303, "ClassPath"=w301, "Template"=w300, "Icon"=w299) -> (w302:T17)
              n163 = in-place-dvr #1(w302) -> ()  [unwired: 2 out]
            }
            n164 = Bundle By Name(cluster=w261, "changeConnection"=w279) -> (w280:T2)
          }
        }
        n165 = Equal?(x=w31, y="Exit") -> (x = y?=w34:bool)
        n166 = Select(t="Error", s=w30, f=w31) -> (s? t:f=w35:string)
      }
      n167 = Unbundle By Name(w12) -> ("changeConnection"=w10:T1, "Cancelled"=w9:bool)
      n168 = call <resource>:"CommonVIs_CloseControlRefs.vi"("Event Registration Refnum"=w11, "ControlRefs"=w22, "error in (no error)"=w14) -> ("error out"=w21:errorcluster)  [unwired: 16 out]
      n169 = call <resource>:"ContextHelp_LeavingDialog.vi"("error in (no error)"=w21) -> ("error out"=w13:errorcluster)  [unwired: 2 in, 16 out]
    }
    frame Error {
    }
  }
  "reference out" <- w4
  "error out" <- w5
  "changeConnection" <- w2
  "cancel" <- w1
